vi "Control Loop Que _NoUSEEEE.vi"(7 "Action Select":enum16{"Initial", "Add", "Release"}(ring)=enum."Release", 8 "error in (no error)":errorcluster, 11 "Control Loop In":T4) -> (0 "error out":errorcluster, 3 "Control Q Out":refnum<queue>)   [LabVIEW 2019]
uses:
  Ctrl/Control Loop_Control.ctl
  Ctrl/Control Loop_Status.ctl
  Ctrl/Process Action Name.ctl
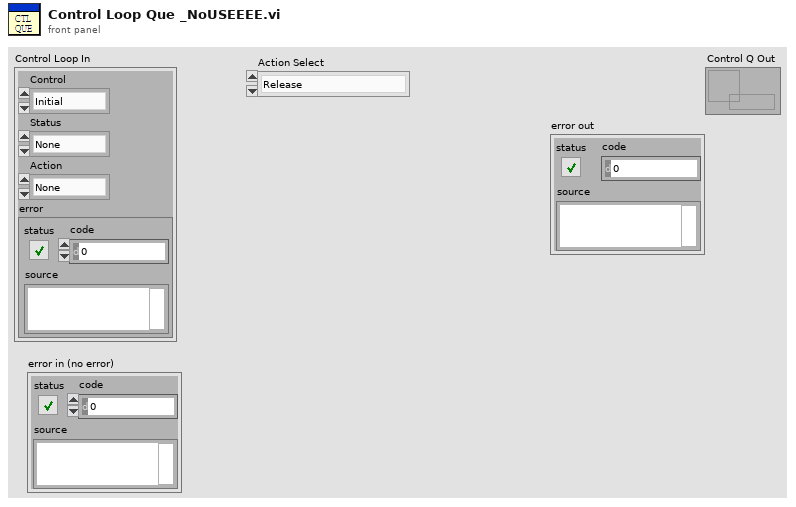
[diagram p1: front panel]
types:
  T1 = typedef "Control Loop_Control.ctl" = enum16{"Initial", "Standby Mode", "Run Mode", "Status", "Exit"}
  T2 = typedef "Control Loop_Status.ctl" = enum16{"None", "Next", "Error", "SafeDoor", "Exit"}
  T3 = typedef "Process Action Name.ctl" = enum16{"None", "*******Initial*******", "*******Check Run*******", "*******Manual*******", "*******Others*******", "*******Exit*******", "Exit"}
  T4 = cluster{"Control":T1, "Status":T2, "Action":T3, "error":errorcluster}
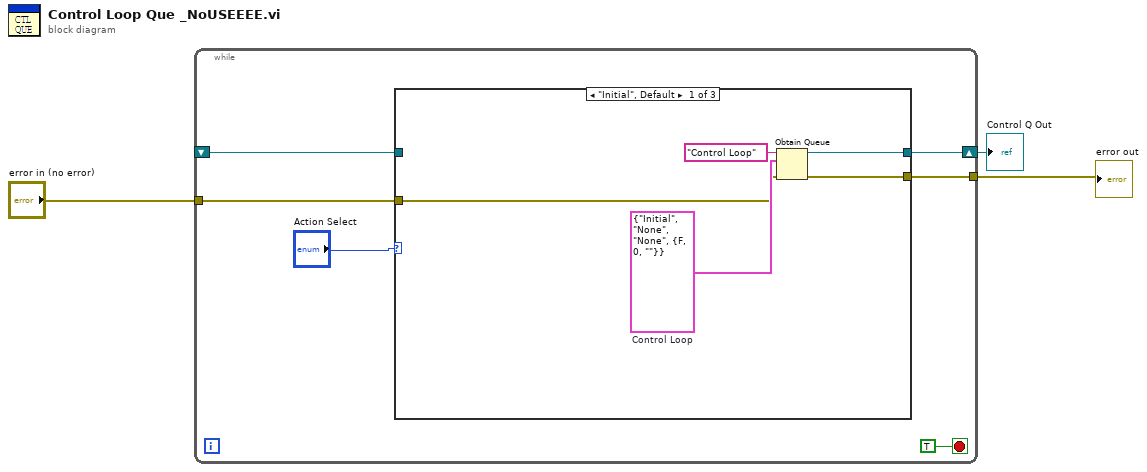
[diagram p0: block diagram]
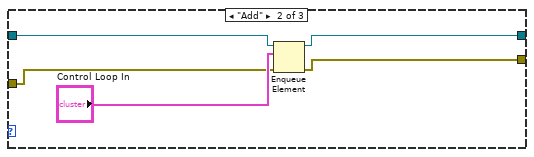
[diagram p2: hidden frame]
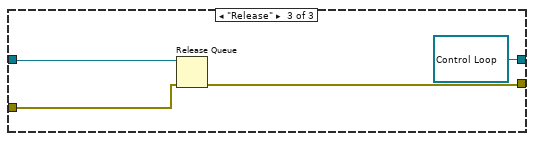
[diagram p3: hidden frame]
diagram:
  n1 = while {
    shift-right: [w9] -> w1
    shift-left: _ -> [w7]
    tunnel: "error in (no error)" -> [w6]
    tunnel: [w5] -> w2
    stop <- TRUE stop-if-true
    n2 = case shown="\"Initial\", Default" "Action Select" {
      tunnel: [w13 w18 refnum<queue> refnum ("queue out")] -> w9
      tunnel: w7 -> [_ w19 w23]
      tunnel: w6 -> [w11 w15 w22]
      tunnel: [w10 w16 w21] -> w5
      frame "Initial", Default {
        w14 = T4 {"Control"=enum."Initial", "Status"=enum."None", "Action"=enum."None", "error"={"status"=FALSE, "code"=0, "source"=""}}  # Control Loop
        n3 = Obtain Queue(name (unnamed)="Control Loop", element data type=w14, error in (no error)=w11) -> (queue out=w13:refnum<queue>, error out=w10:errorcluster)  [unwired: 2 in, 1 out]
      }
      frame "Add" {
        n4 = Enqueue Element(queue=w19, element="Control Loop In", error in (no error)=w15) -> (queue out=w18:refnum<queue>, error out=w16:errorcluster)  [unwired: 1 in, 1 out]
      }
      frame "Release" {
        n5 = Release Queue(queue=w23, error in (no error)=w22) -> (error out=w21:errorcluster)  [unwired: 1 in, 2 out]
      }
    }
  }
  "error out" <- w2
  "Control Q Out" <- w1
